vi "ShowAsynchAndReserve (SubVI).vi"(8 "error constant 2":errorcluster, 10 "Reserve Disk Space in":bool, 11 "Asynchronous Writes in":bool) -> (0 "error constant":errorcluster, 2 "Reserve Disk Space":bool, 3 "Asynchronous Writes":bool)   [LabVIEW 2023]
panel:
  in  "Stop":bool caption="y"
  in  "Continue":bool
  # "If Asynchronous writes is not enabled, I dont know why"
  # "If reserve disk space is not enabled, try running as admin"
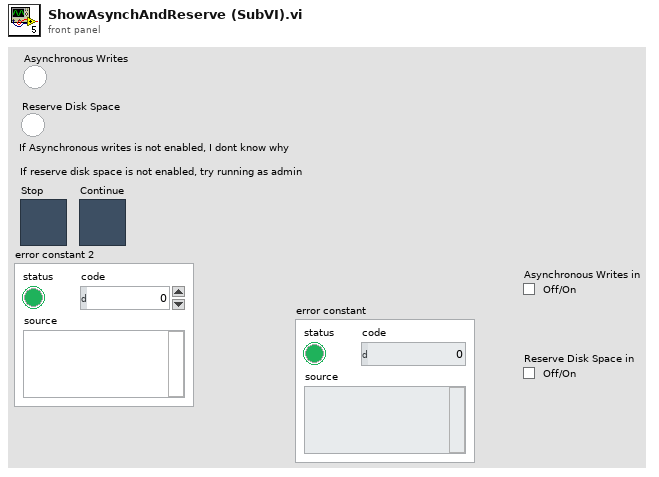
[diagram p1: front panel]
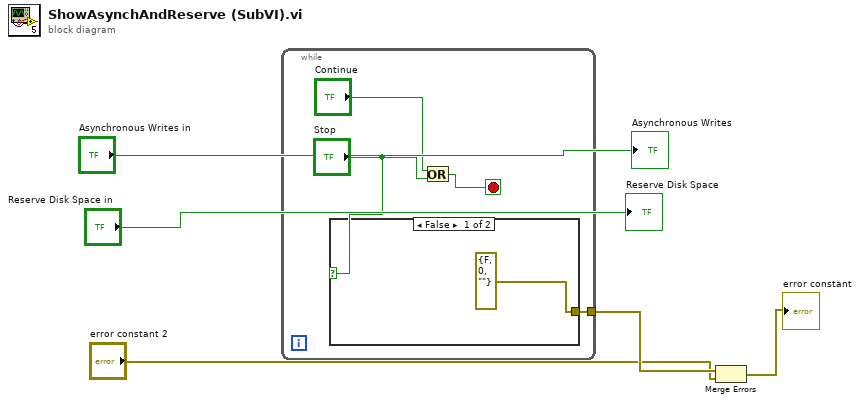
[diagram p0: block diagram]
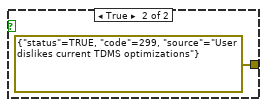
[diagram p2: hidden frame]
diagram:
  n1 = while {
    tunnel: [w6] -> w3
    stop <- w8 stop-if-true
    n2 = case shown="False" "Stop" {
      tunnel: [errorcluster {"status"=FALSE, "code"=0, "source"=""} ("error constant") errorcluster {"status"=TRUE, "code"=299, "source"="User dislikes current TDMS optimizations"} ("error constant")] -> w6
      frame False {
      }
      frame True {
      }
    }
    n3 = Or(x="Continue", y="Stop") -> (x .or. y?=w8:bool)
  }
  n4 = Merge Errors(w3, "error constant 2") -> (→"error constant":errorcluster)
  "Asynchronous Writes" <- "Asynchronous Writes in"
  "Reserve Disk Space" <- "Reserve Disk Space in"
